vi "Attack Enemy.vi"(11 "View in":i32[](array[numeric]) caption="Updated View (-1 team, 0 empty, 1 enemy)") -> (1 "attack direction":T1, 2 "enemy found?":bool, 3 "all enemies":T1[](array[typedef]))   [LabVIEW 2015, in "DS Square.lvlib"]
uses:
  DS Square.lvlib
  Type Defs/Direction Enum.ctl
  Type Defs/SB Type Defs.lvlib
panel:
  # "NW\nN\nNE\nE\nSE\nS\nSW\nW"
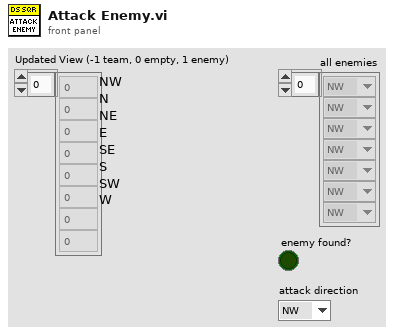
[diagram p1: front panel]
types:
  T1 = typedef "SB Type Defs.lvlib/Direction Enum.ctl" = enum16{"NW", "N", "NE", "E", "SE", "S", "SW", "W"}
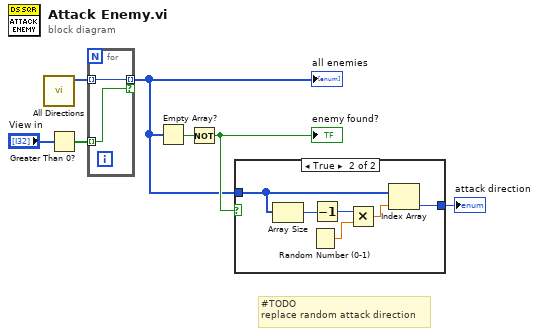
[diagram p0: block diagram]
diagram:
  # "#TODO\nreplace random attack direction"
  n1 = call "All Directions.vi"() -> ("All directions"=w5:T1[])  [unwired: 11 in]
  n2 = Greater Than 0?(x="View in") -> (x > 0?=w6:bool[])
  n3 = for {
    tunnel: w6 -> [w8] mode=indexing
    tunnel: w5 -> [w9] mode=indexing
    tunnel: [w9] -> w2 mode=indexing if=w8
  }
  "all enemies" <- w2
  n4 = Empty Array?(array=w2) -> (empty?=w4:bool)
  n5 = Not(x=w4) -> (.not. x?=w3:bool)
  "enemy found?" <- w3
  n6 = case shown="True" w3 {
    tunnel: w2 -> [_ w11]
    tunnel: [_ w10] -> w1
    frame False {
    }
    frame True {
      n7 = Array Size(array=w11) -> (size(s)=w15:i32)
      n8 = Random Number (0-1)() -> (number: 0 to 1=w13:dbl)
      n9 = Decrement(x=w15) -> (x-1=w14:i32)
      n10 = Multiply(x=w14, y=w13) -> (x*y=w12:dbl)
      n11 = Index Array(array=w11, index=w12) -> (element=w10:T1)
    }
  }
  "attack direction" <- w1
